vi "LauncherFeeder.vi"(2 "Target RPM Feeder":dbl=770.0, 3 "Target RPM Launcher":dbl=3300.0) -> (0 "Feeder RPM":dbl=3319.8279051826034, 1 "Launcher RPM":dbl=3319.8279051826034)   [LabVIEW 2016]
doc: "This example shows how to move a motor connected to an encoder and a wheel, and then read information about the system from an encoder.\n\nThis is an example of how to use feedback (from the encoder) to create an open loop system. If some control method was used, for example using PID, a closed loop system could be created.\n\nThis example expects a USB cable connected from your development PC to the Type B USB Jack (next to the power input) on the roboRIO.\n\nThis example requires the Driver Station to be running with Teleoperated Enabled."
uses:
  <vilib>/gmath/NI_Gmath.lvlib
panel:
  in  "Lower Limit F":dbl=-50.0 format="%#_13g"
  in  "Upper Limit F":dbl=50.0 format="%#_13g"
  in  "Pos Drive Signal F":dbl=0.4
  in  "Neg Drive Signal F":dbl=0.05
  out "Error F":dbl=-19.827905182603445
  out "Encoder Alarm Status F":string="Encoder Moving"
  out "Encoder Direction F":string="Forward"
  in  "Lower Limit L":dbl=-50.0 format="%#_13g"
  in  "Upper Limit L":dbl=50.0 format="%#_13g"
  out "Error L":dbl=-19.827905182603445
  in  "Neg Drive Signal":dbl=0.6
  in  "Pos Drive Signal":dbl=1.0
  out "Loop Time (s)":dbl=0.010378 format="%_6f"
  out "Encoder Alarm Status L":string="Encoder Moving"
  out "Encoder Direction L":string="Forward"
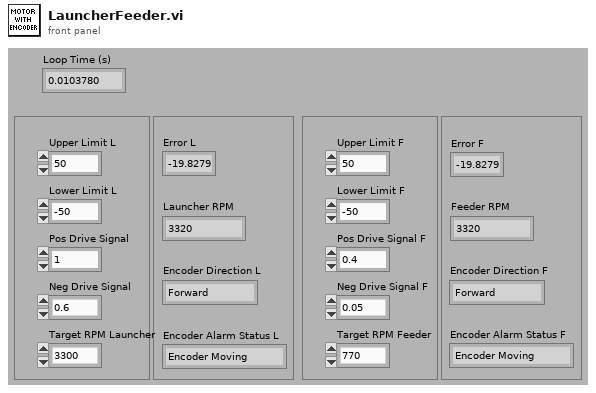
[diagram p1: front panel]
types:
  T1 = typedef "WPI_EncoderDevRef.ctl" = cluster{"DevStatus":errorcluster, "EncoderIndex":T2, "CounterIndex":T3, "DistancePerCount":dbl, "Decoding Type":T4}
  T2 = typedef "FPGA_EncoderIdx.ctl" = enum8{"Enc 0", "Enc 1", "Enc 2", "Enc 3", "Enc 4", "Enc 5", "Enc 6", "Enc 7", "Invalid"}
  T3 = typedef "FPGA_CounterCtrSystemIndex.ctl" = enum8{"Ctr 0", "Ctr 1", "Ctr 2", "Ctr 3", "Ctr 4", "Ctr 5", "Ctr 6", "Ctr 7", "Invalid"}
  T4 = typedef "WPI_EncoderType.ctl" = enum16{"1x", "2x", "4x"}
  T5 = typedef "WPI_MotorControlDeviceRef.ctl" = cluster{"DeviceStatus":errorcluster, "Type":T6, "PWM":cluster{"PWM Channel":T7, "DeadBand":T8}, "CAN":cluster{"Device Number":u8, "SetOutput VI Ref":variant, "GetOutput VI Ref":variant, "Enable VI Ref":variant, "Disable VI Ref":variant, "Data":variant}, "Invert":bool}
  T6 = typedef "WPI_MotorControlType.ctl" = enum16{"PWM", "CAN"}
  T7 = typedef "FPGA_DIOPWMChannel.ctl" = enum8{"PWM 0", "PWM 1", "PWM 2", "PWM 3", "PWM 4", "PWM 5", "PWM 6", "PWM 7", "PWM 8", "PWM 9", "PWM MXP 0", "PWM MXP 1", "PWM MXP 2", "PWM MXP 3", "PWM MXP 4", "PWM MXP 5", "PWM MXP 6", "PWM MXP 7", "PWM MXP 8", "PWM MXP 9", "Invalid"}
  T8 = typedef "WPI_PWMDeadband.ctl" = cluster{"Name":string, "maxPositivePwm":i32, "minPositivePwm":i32, "centerPwm":i32, "maxNegativePwm":i32, "minNegativePwm":i32, "angularRange":u16}
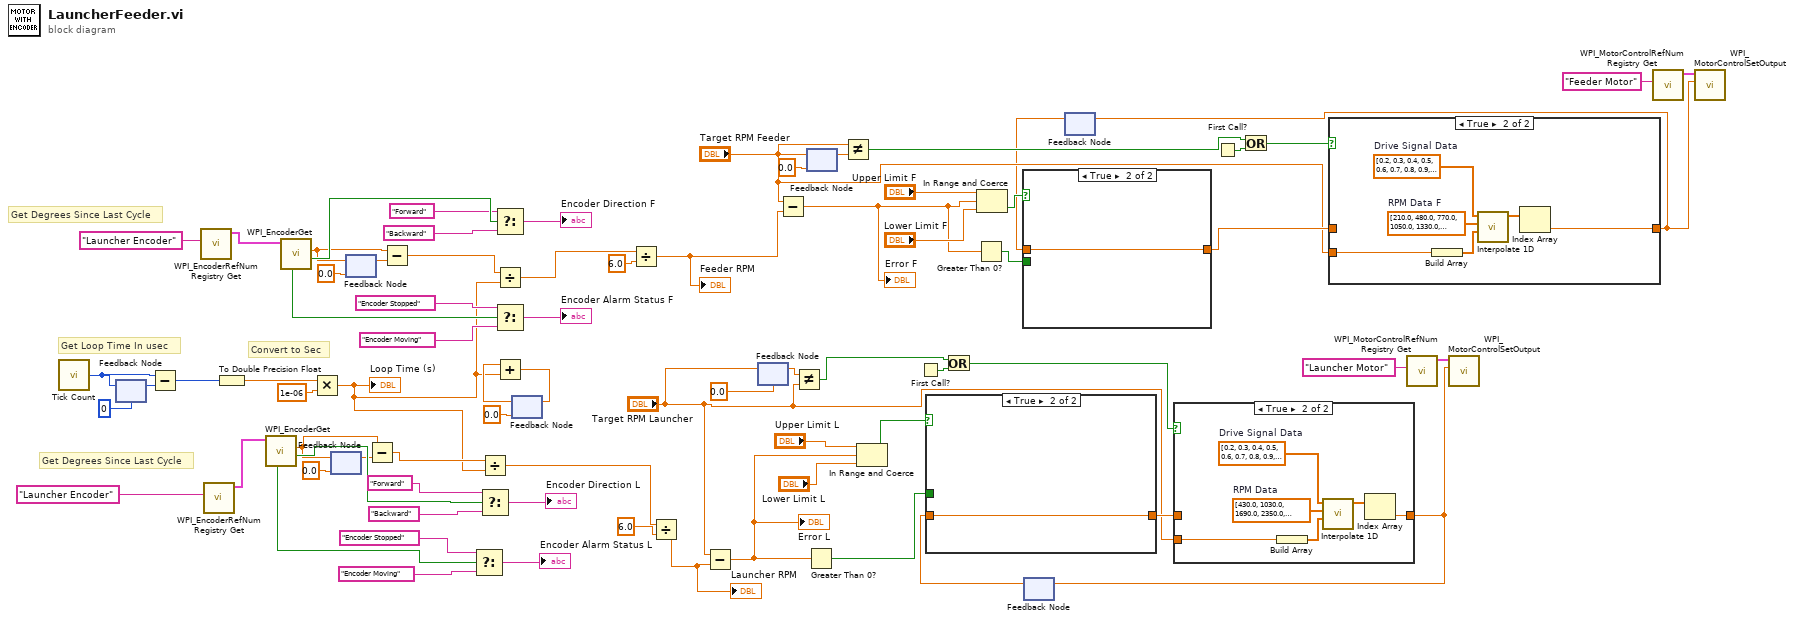
[diagram p0: block diagram]
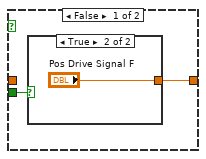
[diagram p3: hidden frame]
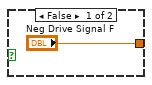
[diagram p4: hidden frame]
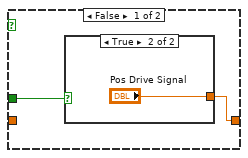
[diagram p6: hidden frame]
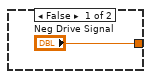
[diagram p7: hidden frame]
diagram:
  # "Get Degrees Since Last Cycle"
  # "Get Degrees Since Last Cycle"
  # "Convert to Sec"
  # "Get Loop Time In usec"
  n1 = call "Tick Count"() -> ("Tick Count(uSec)"=w59:u32)
  n2 = feedback #1(u32 0 ("Tick Count(uSec)")) -> (w58:u32)
  n3 = feedback-in #1(w59) -> ()
  n4 = Subtract(x=w59, y=w58) -> (x-y=w56:u32)
  n5 = call <vilib>:"WPI_EncoderRefNum Registry Get.vi"("refnum name"="Launcher Encoder") -> ("EncoderDevRef"=w70:T1)  [unwired: 9 in, 1 out]
  n6 = call <vilib>:"WPI_EncoderRefNum Registry Get.vi"("refnum name"="Launcher Encoder") -> ("EncoderDevRef"=w69:T1)  [unwired: 9 in, 1 out]
  n7 = To Double Precision Float(number=w56) -> (double precision float=w54:dbl)
  n8 = call <vilib>:"WPI_EncoderGet.vi"("EncoderDevRef"=w69) -> ("Direction"=w66:bool, "Distance"=w40:dbl, "Stopped"=w65:bool)  [unwired: 1 in, 7 out]
  n9 = call <vilib>:"WPI_EncoderGet.vi"("EncoderDevRef"=w70) -> ("Direction"=w37:bool, "Distance"=w18:dbl, "Stopped"=w36:bool)  [unwired: 1 in, 7 out]
  n10 = Multiply(x=w54, y=1e-06) -> (x*y=w17:dbl)
  "Loop Time (s)" <- w17
  n11 = feedback #2(0.0 ("Distance")) -> (w57:dbl)
  n12 = feedback-in #2(w40) -> ()
  n13 = feedback #3(0.0 ("Distance")) -> (w19:dbl)
  n14 = feedback-in #3(w18) -> ()
  n15 = Subtract(x=w40, y=w57) -> (x-y=w53:dbl)
  n16 = Subtract(x=w18, y=w19) -> (x-y=w30:dbl)
  n17 = Select(t="Encoder Stopped", s=w65, f="Encoder Moving") -> (s? t:f=→"Encoder Alarm Status L":string)
  n18 = Divide(x=w53, y=w17) -> (x/y=w52:dbl)
  n19 = Select(t="Forward", s=w66, f="Backward") -> (s? t:f=→"Encoder Direction L":string)
  n20 = Select(t="Forward", s=w37, f="Backward") -> (s? t:f=→"Encoder Direction F":string)
  n21 = Divide(x=w30, y=w17) -> (x/y=w29:dbl)
  n22 = Select(t="Encoder Stopped", s=w36, f="Encoder Moving") -> (s? t:f=→"Encoder Alarm Status F":string)
  n23 = feedback #4(0.0) -> (w51:dbl)
  n24 = Add(x=w51, y=w17) -> (x+y=w50:dbl)
  n25 = feedback-in #4(w50) -> ()
  n26 = Divide(x=w29, y=6.0) -> (x/y=w21:dbl)
  "Feeder RPM" <- w21
  n27 = Divide(x=w52, y=6.0) -> (x/y=w49:dbl)
  "Launcher RPM" <- w49
  n28 = Subtract(x="Target RPM Launcher", y=w49) -> (x-y=w44:dbl)
  "Error L" <- w44
  n29 = feedback #5(0.0 ("Target RPM")) -> (w16:dbl)
  n30 = feedback-in #5("Target RPM Launcher") -> ()
  n31 = Subtract(x="Target RPM Feeder", y=w21) -> (x-y=w24:dbl)
  "Error F" <- w24
  n32 = Not Equal?(x=w16, y="Target RPM Launcher") -> (x != y?=w15:bool)
  n33 = Greater Than 0?(x=w44) -> (x > 0?=w48:bool)
  n34 = feedback #6(0.0 ("Target RPM F")) -> (w14:dbl)
  n35 = feedback-in #6("Target RPM Feeder") -> ()
  n36 = Not Equal?(x="Target RPM Feeder", y=w14) -> (x != y?=w13:bool)
  n37 = In Range and Coerce(upper limit="Upper Limit L", x=w44, lower limit="Lower Limit L") -> (In Range?=w45:bool)  [unwired: 1 out]
  n38 = First Call?() -> (First Call?: T/F=w41:bool)
  n39 = Or(x=w15, y=w41) -> (x .or. y?=w42:bool)
  n40 = Greater Than 0?(x=w24) -> (x > 0?=w28:bool)
  n41 = In Range and Coerce(upper limit="Upper Limit F", x=w24, lower limit="Lower Limit F") -> (In Range?=w25:bool)  [unwired: 1 out]
  n42 = feedback #7() -> (w4:dbl)  [unwired: 1 in]
  n43 = case shown="True" w45 {
    tunnel: w48 -> [w78 _]
    tunnel: [w77 w81] -> w43
    tunnel: w4 -> [_ w81]
    frame False {
      n44 = case shown="True" w78 {
        tunnel: ["Neg Drive Signal" "Pos Drive Signal"] -> w77
        frame False {
        }
        frame True {
        }
      }
    }
    frame True {
    }
  }
  n45 = feedback #8() -> (w1:dbl)  [unwired: 1 in]
  n46 = case shown="True" w25 {
    tunnel: w28 -> [w83 _]
    tunnel: [w82 w86] -> w20
    tunnel: w1 -> [_ w86]
    frame False {
      n47 = case shown="True" w83 {
        tunnel: ["Neg Drive Signal F" "Pos Drive Signal F"] -> w82
        frame False {
        }
        frame True {
        }
      }
    }
    frame True {
    }
  }
  n48 = case shown="True" w42 {
    tunnel: [w87 w89] -> w3
    tunnel: w43 -> [w87 _]
    tunnel: "Target RPM Launcher" -> [_ w88]
    frame False {
    }
    frame True {
      w93 = dbl[] [430.0, 1030.0, 1690.0, 2350.0, 3000.0, 3700.0, 4400.0, 5000.0, 5550.0]  # RPM Data
      w92 = dbl[] [0.2, 0.3, 0.4, 0.5, 0.6, 0.7, 0.8, 0.9, 1.0]  # Drive Signal Data
      n49 = Build Array(w88) -> (w91:dbl[])
      n50 = call <vilib>:"Interpolate 1D.vi"("xi"=w91, "X"=w93, "Y"=w92) -> ("yi"=w90:dbl[])  [unwired: 6 in, 2 out]
      n51 = Index Array(array=w90) -> (element=w89:dbl)  [unwired: 1 in]
    }
  }
  n52 = feedback-in #7(w3) -> ()
  n53 = First Call?() -> (First Call?: T/F=w22:bool)
  n54 = Or(x=w13, y=w22) -> (x .or. y?=w23:bool)
  n55 = case shown="True" w23 {
    tunnel: [w94 w96] -> w2
    tunnel: w20 -> [w94 _]
    tunnel: "Target RPM Feeder" -> [_ w95]
    frame False {
    }
    frame True {
      w100 = dbl[] [210.0, 480.0, 770.0, 1050.0, 1330.0, 1650.0, 1870.0, 2140.0, 2400.0]  # RPM Data F
      w99 = dbl[] [0.2, 0.3, 0.4, 0.5, 0.6, 0.7, 0.8, 0.9, 1.0]  # Drive Signal Data
      n56 = Build Array(w95) -> (w98:dbl[])
      n57 = call <vilib>:"Interpolate 1D.vi"("xi"=w98, "X"=w100, "Y"=w99) -> ("yi"=w97:dbl[])  [unwired: 6 in, 2 out]
      n58 = Index Array(array=w97) -> (element=w96:dbl)  [unwired: 1 in]
    }
  }
  n59 = feedback-in #8(w2) -> ()
  n60 = call <vilib>:"WPI_MotorControlRefNum Registry Get.vi"("refnum name"="Launcher Motor") -> ("MotorControlDevRef"=w75:T5)  [unwired: 9 in, 1 out]
  n61 = call <vilib>:"WPI_MotorControlSetOutput.vi"("Output"=w3, "MotorControlDevRef"=w75) -> ()  [unwired: 2 in, 8 out]
  n62 = call <vilib>:"WPI_MotorControlRefNum Registry Get.vi"("refnum name"="Feeder Motor") -> ("MotorControlDevRef"=w73:T5)  [unwired: 9 in, 1 out]
  n63 = call <vilib>:"WPI_MotorControlSetOutput.vi"("Output"=w2, "MotorControlDevRef"=w73) -> ()  [unwired: 2 in, 8 out]
